vi "Kill.vi"(8 "error in (no error)":errorcluster, 11 "Connection in":refnum<class "Connection.lvclass">) -> (0 "error out":errorcluster, 3 "Connection out":refnum<class "Connection.lvclass">)   [LabVIEW 2022 SP3, in "Connection.lvlib" / "Connection.lvclass"]
uses:
  Connection.lvclass
  C:/Users/jakub/repos/gh/sw4sys/lv-tcp-server-sample/LoggingActor/Source/LoggingActor/LoggingActor/LoggingActor.lvclass
  C:/Program Files (x86)/National Instruments/LabVIEW 2022/vi.lib/ActorFramework/Actor/Actor.lvclass
  _State.ctl
  Connection.lvclass/Connection.ctl
  TcpSocket/Source/TcpSocket/Connection/Connection.lvclass/Connection.ctl
  LoggingActor/Source/LoggingActor/LoggingActor/LoggingActor.lvclass/LoggingActor.ctl
  <vilib>/ActorFramework/Actor/Actor.lvclass/Actor.ctl
  <vilib>/ActorFramework/Message Enqueuer/Message Enqueuer.lvclass/Message Enqueuer.ctl
  LoggingActor/Source/LoggingActor/LoggingActor/Read Logger.vi
  TcpSocket/Source/TcpSocket/Connection/Read Address.vi
  TcpSocket/Source/TcpSocket/Connection/Read Port.vi
  TcpSocket/Source/TcpSocket/Connection/Read Connection.vi
  TcpSocket/Source/TcpSocket/Connection/Read ReadMode.vi
  TcpSocket/Source/TcpSocket/Connection/Read ReadTimeout.vi
  TcpSocket/Source/TcpSocket/Connection/Read WriteTimeout.vi
  <vilib>/ActorFramework/Message Enqueuer/Init from Existing Queue.vi
  <vilib>/ActorFramework/Message Enqueuer/Enqueue.vi
  <vilib>/ActorFramework/Stop Msg/Stop Msg.lvclass
  C:/Program Files (x86)/National Instruments/LabVIEW 2022/vi.lib/ActorFramework/Message/Message.lvclass
  <vilib>/ActorFramework/Message Priority Queue/Priority Enqueue.vi
  TcpSocket/Source/TcpSocket/Connection/Connection.lvclass
  Logger/Source/Logger/Logger.lvclass
  <vilib>/ActorFramework/Message Enqueuer/Message Enqueuer.lvclass
  <vilib>/ActorFramework/Actor/Actor.lvclass
  C:/Users/jakub/repos/gh/sw4sys/lv-tcp-server-sample/TcpServerSample/Source/TcpServerSample/Connection/Connection/Connection.lvclass
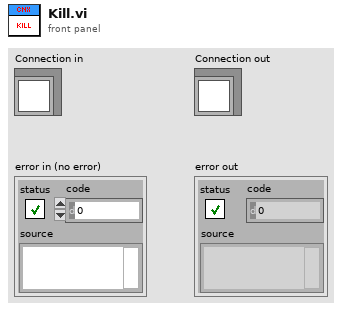
[diagram p1: front panel]
types:
  T1 = typedef "Connection.lvlib/Connection.lvclass/_State.ctl" = enum16{"WaitForInit", "Active", "Dying"}
  T2 = enum16{"Standard", "Buffered", "CRLF", "Immediate"}
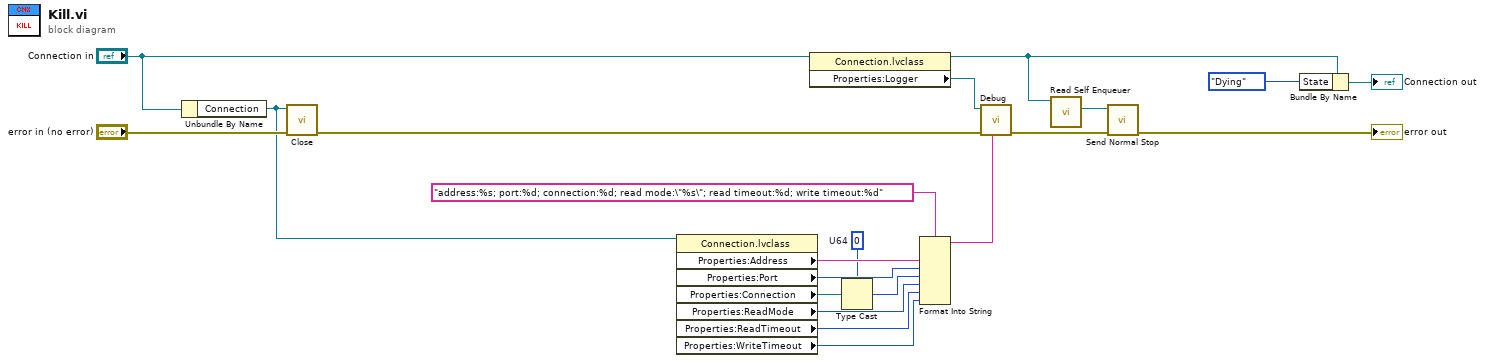
[diagram p0: block diagram]
diagram:
  w11 = u64 0  # U64
  n1 = Unbundle By Name("Connection in") -> ("Connection"=w5:refnum<class "Connection.lvclass">)
  n2 = call-dynamic "Close.vi"("error in (no error)"="error in (no error)", "Connection"=w5) -> ("error out"=w19:errorcluster)  [unwired: 9 in]
  n3 = property class="Connection.lvclass"(reference=w5) -> ("Properties:Address"=w13:string, "Properties:Port"=w12:u16, "Properties:Connection"=w10:refnum<k5>, "Properties:ReadMode"=w8:T2, "Properties:ReadTimeout"=w7:i32, "Properties:WriteTimeout"=w6:i32)  [unwired: 1 in, 2 out]
  n4 = property class="Connection.lvclass"(reference="Connection in") -> (reference out=w4:refnum<class "Connection.lvclass">, "Properties:Logger"=w2:refnum<class "Logger.lvclass">)  [unwired: 1 in, 1 out]
  n5 = Type Cast(type=w11, x=w10) -> (*(type *) &x=w9:u64)
  n6 = Format Into String(format string="address:%s; port:%d; connection:%d; read mode:\"%s\"; read timeout:%d; write timeout:%d", w13, w12, w9, w8, w7, w6) -> (resulting string=w1:string)  [unwired: 2 in, 1 out]
  n7 = call-dynamic "Debug.vi"("Message"=w1, "error in (no error)"=w19, "Logger in"=w2) -> ("error out"=w3:errorcluster)  [unwired: 5 in, 1 out]
  n8 = call <vilib>:"Read Self Enqueuer.vi"("Actor"=w4) -> ("Self Enqueuer"=w20:refnum<class "Message Enqueuer.lvclass">)  [unwired: 10 in]
  n9 = call <vilib>:"Send Normal Stop.vi"("error in (no error)"=w3, "Message Enqueuer"=w20) -> ("error out"=→"error out":errorcluster)  [unwired: 9 in]
  n10 = Bundle By Name(cluster=w4, "State"=_State."Dying") -> (→"Connection out":refnum<class "Connection.lvclass">)
